vi "canon.vi"(6 "T/F":bool, 7 "loop count":dbl, 8 "에러 입력":errorcluster, 9 "spring pull[mm]":dbl, 11 "FPGA VI 참조 입력":refnum<k20>) -> (0 "에러 출력":errorcluster, 2 "직동_dir":bool, 3 "FPGA VI 참조 출력":refnum<k20>)   [LabVIEW 2019]
uses:
  <vilib>/Utility/error.llb/Error Cluster From Error Code.vi
  <vilib>/rvi/errors/niLvFpgaAdjustHostInterfaceError.vi
  <vilib>/rvi/interface/nirviReadWriteControl/nirviReadWriteControl.xnode
  <vilib>/rvi/interface/Simulation/niFpgaSimulationCallBeginRW.vi
  NiFpgaLv.dll
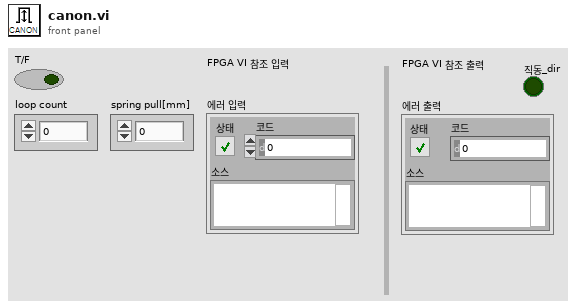
[diagram p1: front panel]
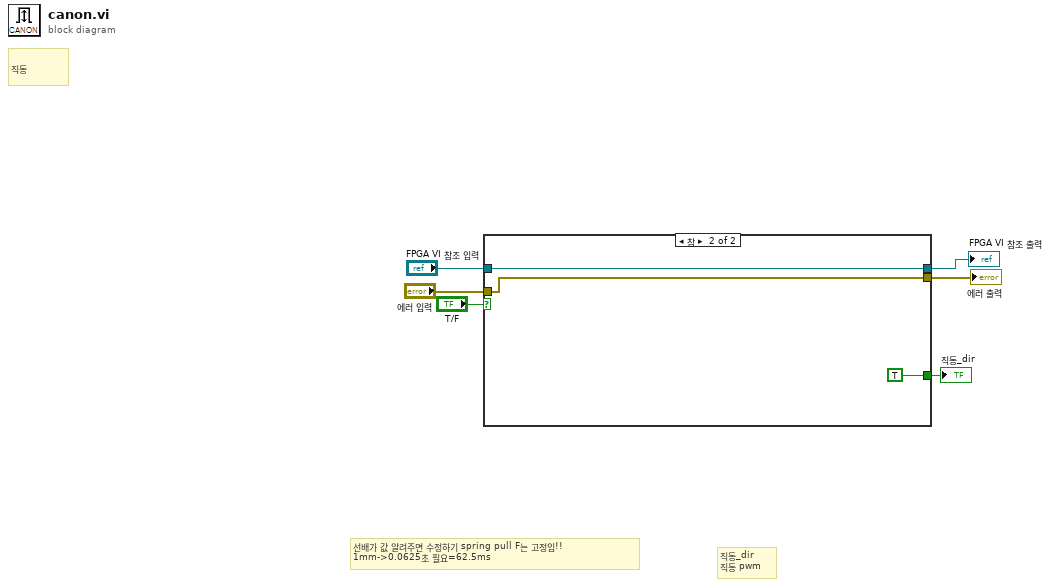
[diagram p0: block diagram]
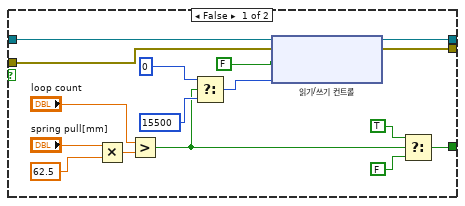
[diagram p2: hidden frame]
diagram:
  # "직동_dir\n직동 pwm"
  # "선배가 값 알려주면 수정하기 spring pull F는 고정임!!\n1mm->0.0625초 필요=62.5ms"
  # "직동"
  n1 = case shown="참" "T/F" {
    tunnel: [w18 TRUE ("직동_dir")] -> w5
    tunnel: [w12 w24] -> w4
    tunnel: [w11 w23] -> w3
    tunnel: "FPGA VI 참조 입력" -> [w8 w24]
    tunnel: "에러 입력" -> [w7 w23]
    frame False {
      n2 = Multiply(x="spring pull[mm]", y=62.5) -> (x*y=w21:dbl)
      n3 = Greater?(x="loop count", y=w21) -> (0:w13:bool)
      n4 = Select(t=0 ("직동_pwm input"), s=w13, f=15500 ("직동_pwm input")) -> (s? t:f=w9:i32)
      n5 = xnode "읽기/쓰기 컨트롤"("FPGA VI 참조 입력"=w8, "에러 입력"=w7, "직동_dir"=FALSE, "직동_pwm input"=w9) -> ("FPGA VI 참조 출력"=w12:refnum<k20>, "에러 출력"=w11:errorcluster)
      n6 = Select(t=TRUE ("직동_dir"), s=w13, f=FALSE ("직동_dir")) -> (s? t:f=w18:bool)
    }
    frame True {
    }
  }
  "직동_dir" <- w5
  "FPGA VI 참조 출력" <- w4
  "에러 출력" <- w3
